vi "Read Item Tag.vi"(8 "error in (no error)":errorcluster, 11 "TreeItemOpenMsg in":refnum<class "TreeItemOpenMsg.lvclass">) -> (0 "error out":errorcluster, 2 "Item Tag":string, 3 "TreeItemOpenMsg out":refnum<class "TreeItemOpenMsg.lvclass">)   [LabVIEW 2020, in "ActorEvents.lvlib" / "TreeItemOpenMsg.lvclass"]
uses:
  <vilib>/gpm_packages/@cs/mva-viewable/Source/ActorEvents/IEventAggregator Messages/TreeItemOpenMsg/TreeItemOpenMsg.lvclass
  <vilib>/gpm_packages/@cs/mva-viewable/Source/ActorEvents/IEventAggregator Messages/TreeItemOpenMsg/TreeItemOpenMsg.lvclass/TreeItemOpenMsg.ctl
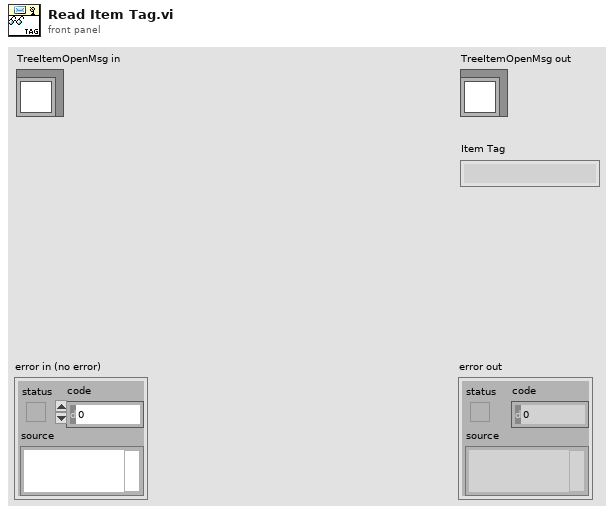
[diagram p1: front panel]
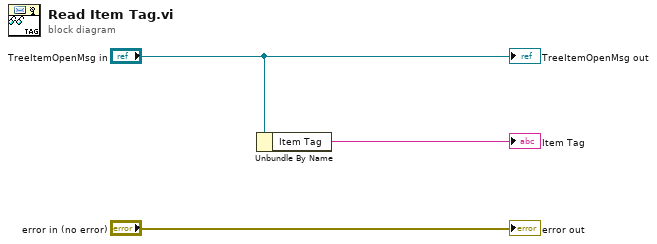
[diagram p0: block diagram]
diagram:
  n1 = Unbundle By Name("TreeItemOpenMsg in") -> ("Item Tag"=→"Item Tag":string)
  "error out" <- "error in (no error)"
  "TreeItemOpenMsg out" <- "TreeItemOpenMsg in"
